vi "session_callback_send_function.vi"(8 "error in (no error)":errorcluster, 9 "flags":i32, 10 "buffer":u8[](array[numeric]), 11 "socket":u64) -> (0 "error out":errorcluster, 2 "bytes send":i64)   [LabVIEW 2013]
doc: "Called when libssh2 wants to send data on the connection.\n\n<B>socket</B> is the socket to write to.\n<B>buffer</B> is the data to send.\n<B>flags</B> are the flags that would have been used by a send() call.\n\nReturns the number of bytes sent."
uses:
  ws2_32.dll
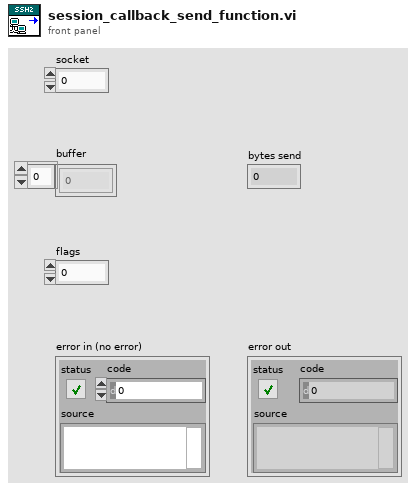
[diagram p1: front panel]
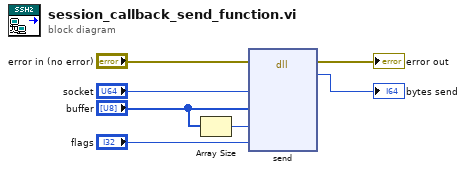
[diagram p0: block diagram]
diagram:
  n1 = Array Size(array="buffer") -> (size(s)=w5:i32)
  n2 = dll-call lib="ws2_32.dll" fn="send"(error in="error in (no error)", "s"="socket", "buf"="buffer", "len"=w5, "flags"="flags") -> (error out=→"error out":errorcluster, "return type"=→"bytes send":i32)  [unwired: 6 in, 1 out]
